vi "create global stop.vi"(11 "Template in":refnum<class "Template.lvclass">) -> (0 "error out":errorcluster, 3 "Template out":refnum<class "Template.lvclass">)   [LabVIEW 2020, in "Template.lvlib" / "Template.lvclass"]
uses:
  Template.lvclass
  typedefs/global stop.ctl
  Template.lvclass/Template.ctl
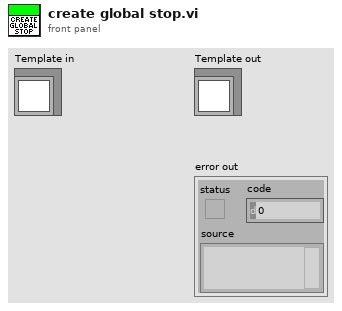
[diagram p1: front panel]
types:
  T1 = typedef "Template.lvlib/Template.lvclass/global stop.ctl" = cluster{"Global Stop Notifier":refnum<notifier>, "Global Stop Event":refnum<user-event>}
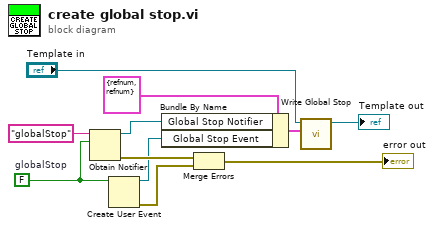
[diagram p0: block diagram]
diagram:
  w8 = FALSE  # globalStop
  n1 = Obtain Notifier(name (unnamed)="globalStop", notification data type=w8) -> (notifier out=w5:refnum<notifier>, error out=w9:errorcluster)  [unwired: 2 in, 1 out]
  n2 = Create User Event(user event datatype=w8) -> (user event=w4:refnum<user-event>, error out=w1:errorcluster)  [unwired: 1 in]
  n3 = Bundle By Name(cluster=T1 {"Global Stop Notifier"=refnum, "Global Stop Event"=refnum} ("Global Stop"), "Global Stop Notifier"=w5, "Global Stop Event"=w4) -> (w3:T1)
  n4 = Merge Errors(w9, w1) -> (→"error out":errorcluster)
  n5 = call "Write Global Stop.vi"("Global Stop"=w3, "Template in"="Template in") -> ("Template out"=→"Template out":refnum<class "Template.lvclass">)  [unwired: 9 in]
